vi "daq.io Get Time Series Example.vi"(8 "error in":errorcluster) -> (0 "error out":errorcluster)   [LabVIEW 2013, in "daqio minimal.lvlib"]
doc: "This interactive example demonstrates how to retrieve time series data stored on daq.io in your LabVIEW environment. After connecting, select the device to view data for. Choose a channel to view, select a start and end time to filter data for and choose a time resolution. \n\nMonthly Rollups are very small documents that contain the hourly averages of all measured values.\nDaily Rollups are medium sized documents that contain the measured values averaged to minute data. \nThe Hourly Rollups are documents that store the original resolution with a maximum resolution of 1 Hz. \n\nClick \"Download Data\" to view the selected time frame. \n\nIf Waveform data has been stored on a channel, once you select a channel and filter the start end end time, all existing Waveform documents will be listed below the charting area. Double-click a waveform to download and display it."
uses:
  daqio minimal.lvlib
  _typedefs/exmpl_overlay_mask.ctl
  _typedefs/daqio-rollups-resolution.ctl
  _typedefs/download-2-button.ctl
  _typedefs/daqio-Credentials.ctl
  _typedefs/daqio-Type.ctl
  <vilib>/httpClient/ClientHandle.ctl
  _typedefs/daqio-Device-Specifier.ctl
  <vilib>/Platform/browser.llb/Open URL in Default Browser (string).vi
  <vilib>/httpClient/LabVIEWHTTPClient.lvlib
panel:
  out "overlay mask":T1
  in  "Waveforms":i32(listbox) caption="Waveforms (double-click to view)"
  out "Wfm Graph":waveform(dbl)[](graph) caption="Waveform Graph"
  out "Timeseries Data Graph":cluster{"timestamp":timestamp, "value":dbl}[](graph)
  out "Waveform":string
  in  "Device":u16(ring) items=["DESKTOP_7UDDDR9_LOCALDOMAIN"]
  in  "Download Time Series":T2
  in  "time resolution":T3
  in  "End Time":timestamp
  in  "Start Time":timestamp
  out "selected Channel":string
  in  "Channels":i32(listbox)
  out "Log":string[](array[string])
  in  "Stop":bool
  out "connected to daq.io":bool
  in  "Sign up link":bool caption="Boolean"
  out "Device Key":string
  in  "Log On":bool
  in  "User Name (your email)":string
  in  "Password":string
  # "Get your free account at daq.io first: sign up at"
  # "This Machine"
  # "Select Device to Read Data From"
  # "Device Channel Data"
  # "Select Data Channel"
  # "Specifiy Data to Be Viewed"
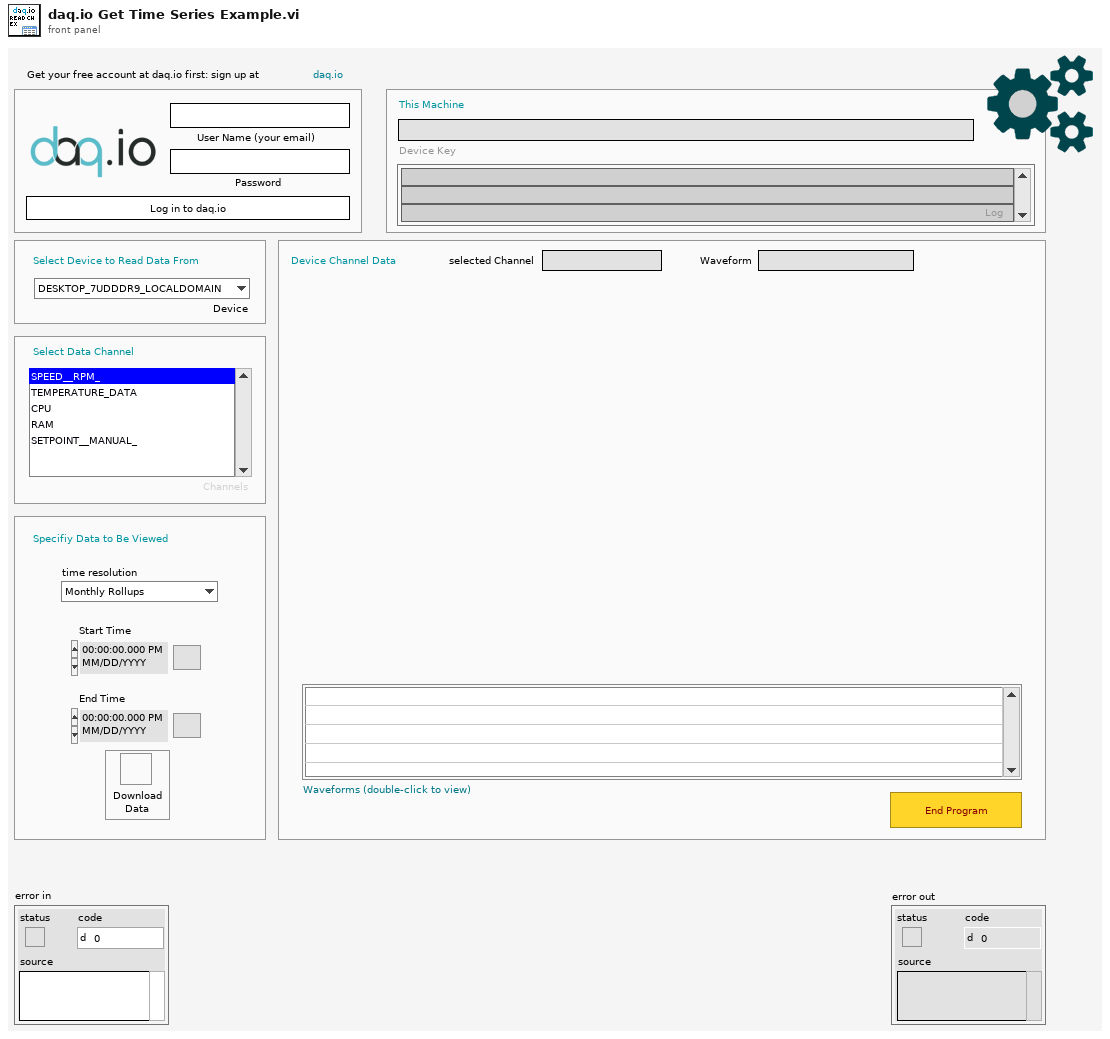
[diagram p1: front panel]
types:
  T1 = typedef "daqio minimal.lvlib/exmpl_overlay_mask.ctl" = bool
  T2 = typedef "daqio minimal.lvlib/download-2-button.ctl" = bool
  T3 = typedef "daqio minimal.lvlib/daqio-rollups-resolution.ctl" = enum16{"Monthly Rollups", "Daily Rollups", "Hourly Rollups (seconds)"}
  T4 = typedef "daqio minimal.lvlib/daqio-Credentials.ctl" = cluster{"User Name (email)":string, "Password":string}
  T5 = typedef "daqio minimal.lvlib/daqio-Device-Specifier.ctl" = cluster{"Device Key":string, "Device Label":string}
  T6 = typedef "daqio minimal.lvlib/daqio-Type.ctl" = cluster{"daq.io ref":T7, "daq.io API Base":string, "Device Key":string, "Account ID":string, "online":bool, "SSL":bool}
  T7 = typedef "LabVIEWHTTPClient.lvlib/ClientHandle.ctl" = refnum<k1>
  T8 = typedef "daqio minimal.lvlib/daqio-Device.ctl" = cluster{"id":string, "label":string, "key":string, "channels":T9[], "tags":cluster{"key":string, "value":string}[], "events":cluster{"id":string, "key":string, "label":string}[], "files":string[], "permissions":cluster{"write":string[], "read":string[]}, "dashboard":string}
  T9 = typedef "daqio minimal.lvlib/daqio-Channels.ctl" = cluster{"key":string, "label":string, "data_type":string, "id":string}
  T10 = typedef "daqio minimal.lvlib/daqio-read-waveform-JSON-header-time.ctl" = cluster{"id":string, "label":string, "channel":string, "device":string, "start_time":timestamp}
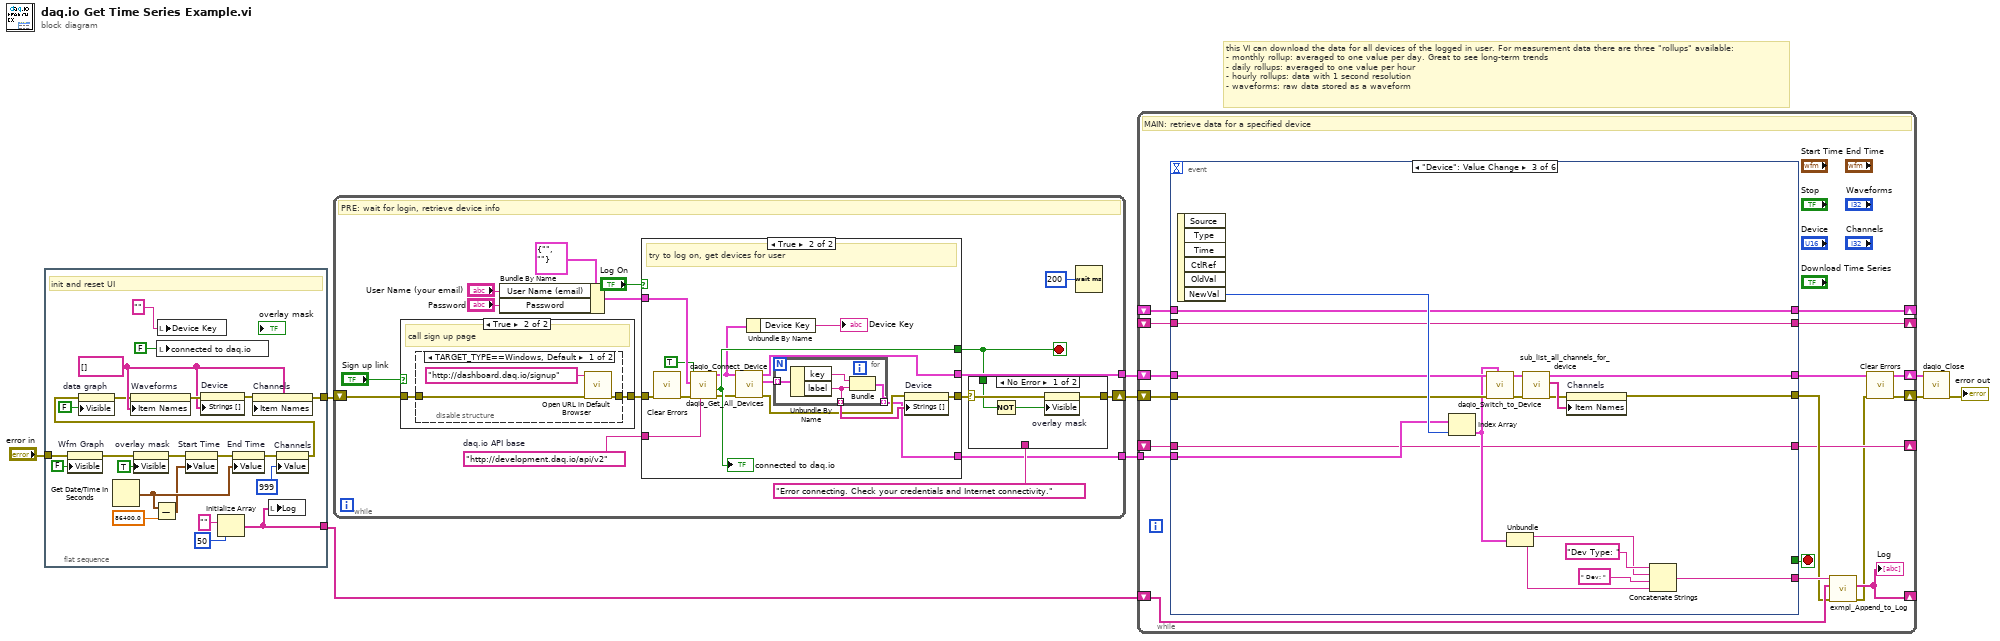
[diagram p0: block diagram]
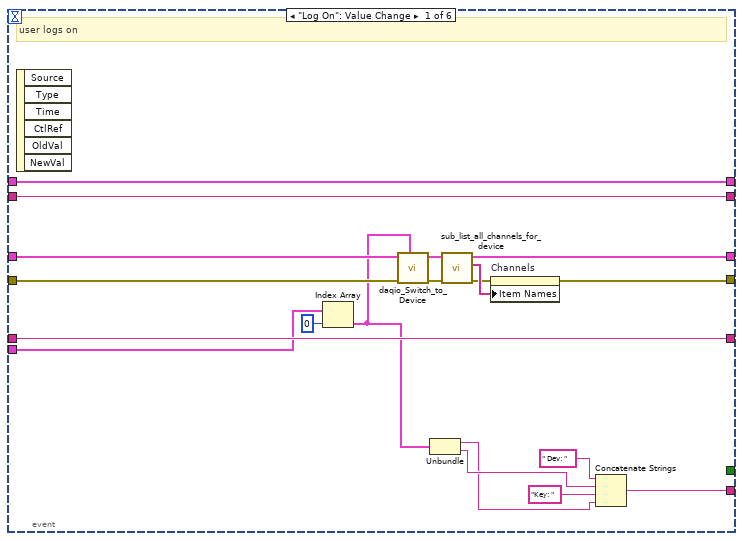
[diagram p2: hidden frame]
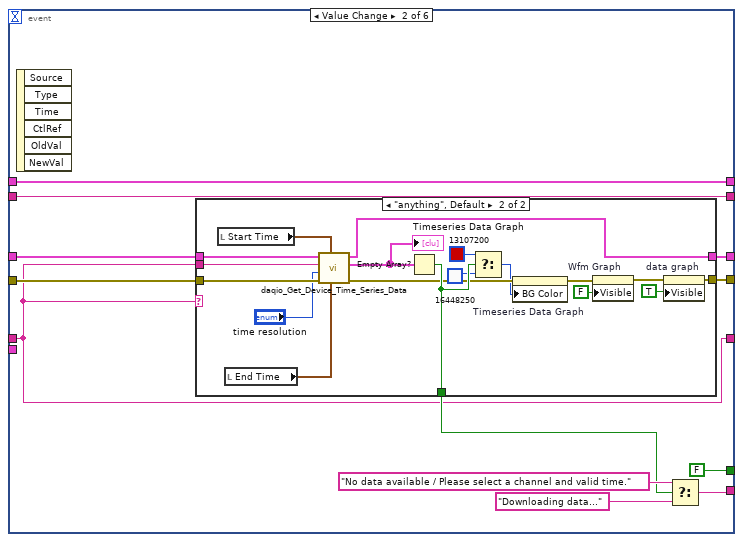
[diagram p3: hidden frame]
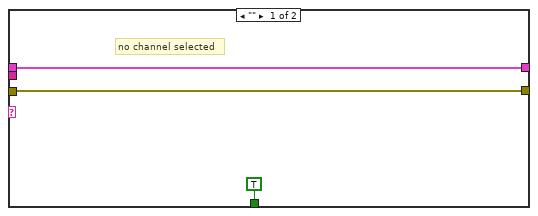
[diagram p4: hidden frame]
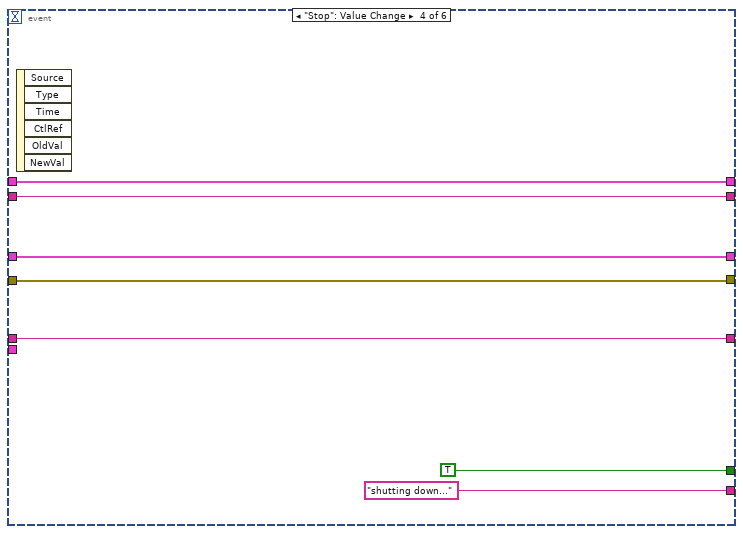
[diagram p5: hidden frame]
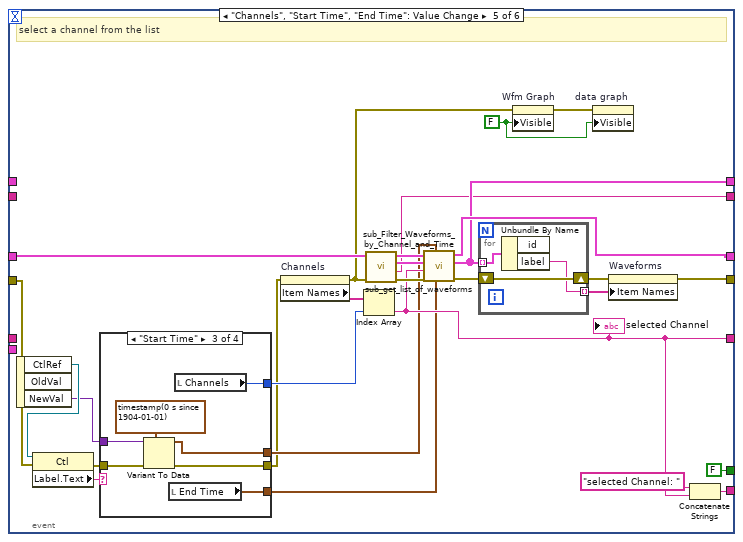
[diagram p6: hidden frame]
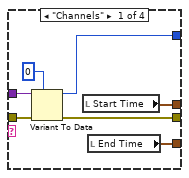
[diagram p7: hidden frame]
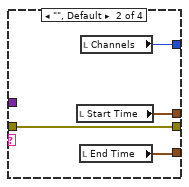
[diagram p8: hidden frame]
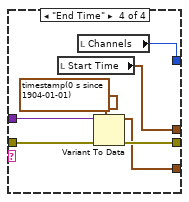
[diagram p9: hidden frame]
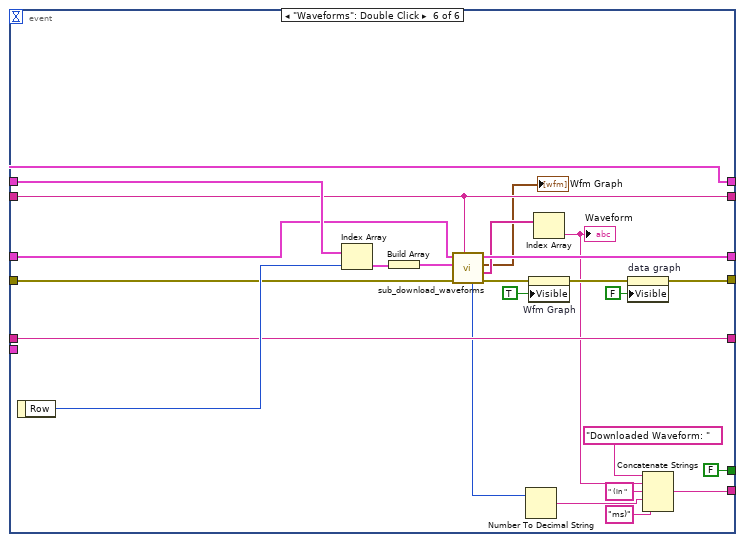
[diagram p10: hidden frame]
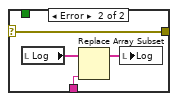
[diagram p11: hidden frame]
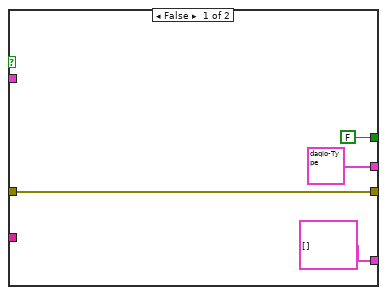
[diagram p14: hidden frame]
diagram:
  # "this VI can download the data for all devices of the logged in user. For measurement data there are three \"rollups\" available: \n- monthly rollup: averaged to one value per day. Great to see long-term trends\n- daily rollups: averaged to one value per hour\n- hourly rollups: data with 1 second resolution\n- waveforms: raw data stored as a waveform"
  n1 = flat-sequence {
    tunnel: [w18] -> w7
    tunnel: "error in" -> [w15]
    tunnel: [w27] -> w3
    frame #0 {
      w16 = string[] [] ("Item Names")
      # "init and reset UI"
      n2 = property on="Wfm Graph" class="WFGraph (strict)"(error in=w15, "Visible"=FALSE) -> (error out=w13:errorcluster)  [unwired: 1 in, 1 out]
      n3 = Get Date/Time In Seconds() -> (seconds since 1Jan1904=w24:timestamp)
      n4 = property on="overlay mask" class="Bool (strict)"(error in=w13, "Visible"=TRUE) -> (error out=w26:errorcluster)  [unwired: 1 in, 1 out]
      n5 = Subtract(x=w24, y=86400.0) -> (x-y=w22:timestamp)
      n6 = local write "connected to daq.io"(FALSE ("connected to daq.io")) -> ()
      n7 = local write "Device Key"("" ("log")) -> ()
      n8 = property on="Start Time" class="AbsTime (strict)"(error in=w26, "Value"=w22) -> (error out=w25:errorcluster)  [unwired: 1 in, 1 out]
      n9 = Initialize Array("" ("log"), 50 ("dimension size")) -> (w27:string[])
      n10 = property on="End Time" class="AbsTime (strict)"(error in=w25, "Value"=w24) -> (error out=w20:errorcluster)  [unwired: 1 in, 1 out]
      n11 = local write "Log"(w27) -> ()
      n12 = property on="Channels" class="LstBox (strict)"(error in=w20, "Value"=999 ("Channels")) -> (error out=w12:errorcluster)  [unwired: 1 in, 1 out]
      n13 = property on="data graph" class="XYGraph (strict)"(error in=w12, "Visible"=FALSE) -> (error out=w11:errorcluster)  [unwired: 1 in, 1 out]
      n14 = property on="Waveforms" class="LstBox (strict)"(error in=w11, "Item Names"=w16) -> (error out=w17:errorcluster)  [unwired: 1 in, 1 out]
      n15 = property on="Device" class="Ring (strict)"(error in=w17, "Strings []"=w16) -> (error out=w19:errorcluster)  [unwired: 1 in, 1 out]
      n16 = property on="Channels" class="LstBox (strict)"(error in=w19, "Item Names"=w16) -> (error out=w18:errorcluster)  [unwired: 1 in, 1 out]
    }
  }
  n17 = while {
    shift-right: [w35] -> w5
    shift-left: w7 -> [w41]
    tunnel: [w43] -> w6
    tunnel: [w34] -> w2
    stop <- w33 stop-if-true
    w38 = "http://development.daq.io/api/v2"  # daq.io API base
    # "PRE: wait for login, retrieve device info"
    n18 = case shown="True" "Sign up link" {
      tunnel: w41 -> [w57 w59]
      tunnel: [w57 w58] -> w40
      frame False {
      }
      frame True {
        # "call sign up page"
        n19 = disable-structure shown="TARGET_TYPE==Windows, Default" {
          disable-tunnel: w59 -> [w61 w63]
          disable-tunnel: [w60 w63] -> w58
          frame condition #0 (active) {
            n20 = call-poly <vilib>:"Open URL in Default Browser.vi"("error in (no error)"=w61, "URL"="http://dashboard.daq.io/signup") -> ("error out"=w60:errorcluster)  [unwired: 4 in, 1 out]
          }
          frame condition #1 {
          }
        }
      }
    }
    n21 = Bundle By Name(cluster=T4 {"User Name (email)"="", "Password"=""} ("daq.io Credentials"), "User Name (email)"="User Name (your email)", "Password"="Password") -> (w42:T4)
    n22 = case shown="True" "Log On" {
      tunnel: [T6 {"daq.io ref"=refnum, "daq.io API Base"="http://dashboard.daq.io/api/v1", "Device Key"="", "Account ID"="", "online"=FALSE, "SSL"=FALSE} ("daq.io type out") w72] -> w43
      tunnel: [w65 w76] -> w36
      tunnel: w40 -> [w65 w82]
      tunnel: w38 -> [_ w81]
      tunnel: w42 -> [_ w80]
      tunnel: [FALSE ("connected successfully?") w79] -> w33
      tunnel: [T5[] [] ("List of Devices") w68] -> w34
      frame False {
      }
      frame True {
        # "try to log on, get devices for user"
        n23 = call <vilib>:"Clear Errors.vi"("error in (no error)"=w82) -> ("error out"=w78:errorcluster)  [unwired: 6 in]
        n24 = call "daqio_Connect_Device.vi"("daq.io API base"=w81, "error in (no error)"=w78, "Credentials"=w80, "Use System Status Event?"=TRUE) -> ("error out"=w75:errorcluster, "connected successfully?"=w79:bool, "daq.io type out"=w74:T6)  [unwired: 5 in]
        "connected to daq.io" <- w79
        n25 = call "daqio_Get_All_Devices.vi"("error in"=w75, "daq.io type in"=w74) -> ("error out"=w70:errorcluster, "Devices"=w73:T8[], "daq.io type out"=w72:T6)  [unwired: 7 in]
        n26 = Unbundle By Name(w74) -> ("Device Key"=→"Device Key":string)
        n27 = for {
          tunnel: w73 -> [w86] mode=indexing
          tunnel: [w85] -> w71 mode=indexing
          tunnel: [w83] -> w68 mode=indexing
          n28 = Unbundle By Name(w86) -> ("key"=w84:string, "label"=w85:string)
          n29 = Bundle("key"=w84, "label"=w85) -> (w83:cluster{"key":string, "label":string})  [unwired: 1 in]
        }
        n30 = property on="Device" class="Ring (strict)"(error in=w70, "Strings []"=w71) -> (error out=w76:errorcluster)  [unwired: 1 in, 1 out]
      }
    }
    n31 = case shown="No Error" w36 {
      selector: w36 -> [w51 w53]
      tunnel: "Error connecting. Check your credentials and Internet connectivity." ("new element/subarray") -> [_ w54]
      tunnel: [w52 w53] -> w35
      tunnel: w33 -> [w50 _]
      frame No Error {
        n32 = Not(x=w50) -> (.not. x?=w49:bool)
        n33 = property on="overlay mask" class="Bool (strict)"(error in=w51, "Visible"=w49) -> (error out=w52:errorcluster)  [unwired: 1 in, 1 out]
      }
      frame Error {
        n34 = local read "Log"() -> (w56:string[])
        n35 = Replace Array Subset(array=w56, new element=w54) -> (w55:string[])  [unwired: 1 in]
        n36 = local write "Log"(w55) -> ()
      }
    }
    n37 = Wait (ms)(milliseconds to wait=u32 200) -> ()  [unwired: 1 out]
  }
  n38 = while {
    shift-right: [w93] -> w9
    shift-left: w5 -> [w99]
    shift-right: [w96] -> w4
    shift-left: w6 -> [w98]
    shift-right: [w103] -> _
    shift-left: w3 -> [w101]
    shift-right: [w95] -> _
    shift-left: _ -> [w94]
    tunnel: w2 -> [w91]
    shift-right: [w90] -> _
    shift-left: _ -> [w89]
    shift-right: [w88] -> _
    shift-left: _ -> [w87]
    stop <- w102 stop-if-true
    # "MAIN: retrieve data for a specified device"
    n39 = event shown="[2] \"Device\": Value Change" {
      selector: _ -> [_ _ _ _ _ _]
      dyn-events: _ -> [_ _ _ _ _ _]
      timeout: _ -> [_ _ _ _ _ _]
      tunnel: [_ FALSE _ TRUE FALSE FALSE] -> w102
      tunnel: [w111 w130 w159 "shutting down..." w206 w242] -> w100
      tunnel: w99 -> [w116 w134 w171 w178 w188 w257]
      tunnel: w98 -> [w117 w133 w172 w177 w205 w256]
      tunnel: [w112 w126 w165 w178 w198 w252] -> w97
      tunnel: [w113 w127 w166 w177 w197 w254] -> w96
      tunnel: [w122 w123 w156 w179 w201 w246] -> w95
      tunnel: w94 -> [w122 w123 w156 w179 _ w246]
      tunnel: w91 -> [w114 _ w173 _ _ _]
      tunnel: [w110 w125 w158 w176 w195 w260] -> w90
      tunnel: w89 -> [w110 w125 w158 w176 _ w260]
      tunnel: [w109 w124 w157 w175 w194 w255] -> w88
      tunnel: w87 -> [w109 w124 w157 w175 _ w255]
      event "Log On": Value Change {
        # "user logs on"
        n40 = event-data() -> ()  [unwired: 1 in, 6 out]
        n41 = Index Array(array=w114, index=0) -> (element=w108:T5)
        n42 = call "daqio_Switch_to_Device.vi"("Device to switch to"=w108, "error in (no error)"=w116, "daq.io type in"=w117) -> ("error out"=w120:errorcluster, "daq.io type out"=w121:T6)  [unwired: 7 in]
        n43 = Unbundle(w108) -> ("Device Key"=w104:string, "Device Label"=w106:string)
        n44 = call "sub_list_all_channels_for_device.vi"("error in (no error)"=w120, "daq.io type in"=w121) -> ("error out"=w118:errorcluster, "List of Channel Keys"=w119:string[], "daq.io type out"=w113:T6)  [unwired: 7 in]
        n45 = property on="Channels" class="LstBox (strict)"(error in=w118, "Item Names"=w119) -> (error out=w112:errorcluster)  [unwired: 1 in, 1 out]
        n46 = Concatenate Strings(" Dev: ", w106, "Key: " ("string"), w104) -> (w111:string)
      }
      event Value Change {
        n47 = event-data() -> ()  [unwired: 1 in, 6 out]
        n48 = case shown="\"anything\", Default" w123 {
          tunnel: w134 -> [w136 w155]
          tunnel: w133 -> [w135 w154]
          tunnel: w123 -> [_ w153]
          tunnel: [TRUE ("empty?") w150] -> w129
          tunnel: [w135 w148] -> w127
          tunnel: [w136 w141] -> w126
          frame "" {
            # "no channel selected"
          }
          frame "anything", Default {
            n49 = local read "Start Time"() -> (w138:timestamp)
            n50 = local read "End Time"() -> (w139:timestamp)
            n51 = call "daqio_Get_Device_Time_Series_Data.vi"("End Time"=w139, "Start Time"=w138, "error in (no error)"=w155, "time resolution"="time resolution", "Channel Key"=w153, "daq.io type in"=w154) -> ("error out"=w149:errorcluster, "Datapoints out"=w151:cluster{"timestamp":timestamp, "value":dbl}[], "daq.io type out"=w148:T6)  [unwired: 3 in]
            "Timeseries Data Graph" <- w151
            n52 = Empty Array?(array=w151) -> (empty?=w150:bool)
            n53 = Select(t=u32 13107200, s=w150, f=u32 16448250) -> (s? t:f=w146:u32)
            n54 = property on="Timeseries Data Graph" class="XYGraph (strict)"(error in=w149, "BG Color"=w146) -> (error out=w144:errorcluster)  [unwired: 1 in, 1 out]
            n55 = property on="Wfm Graph" class="WFGraph (strict)"(error in=w144, "Visible"=FALSE) -> (error out=w140:errorcluster)  [unwired: 1 in, 1 out]
            n56 = property on="data graph" class="XYGraph (strict)"(error in=w140, "Visible"=TRUE) -> (error out=w141:errorcluster)  [unwired: 1 in, 1 out]
          }
        }
        n57 = Select(t="No data available / Please select a channel and valid time.", s=w129, f="Downloading data...") -> (s? t:f=w130:string)
      }
      event "Device": Value Change {
        n58 = event-data() -> ("NewVal"=w174:u16)  [unwired: 1 in, 5 out]
        n59 = Index Array(array=w173, index=w174) -> (element=w162:T5)
        n60 = call "daqio_Switch_to_Device.vi"("Device to switch to"=w162, "error in (no error)"=w171, "daq.io type in"=w172) -> ("error out"=w169:errorcluster, "daq.io type out"=w170:T6)  [unwired: 7 in]
        n61 = Unbundle(w162) -> ("Device Key"=w161:string, "Device Label"=w160:string)
        n62 = call "sub_list_all_channels_for_device.vi"("error in (no error)"=w169, "daq.io type in"=w170) -> ("error out"=w167:errorcluster, "List of Channel Keys"=w168:string[], "daq.io type out"=w166:T6)  [unwired: 7 in]
        n63 = property on="Channels" class="LstBox (strict)"(error in=w167, "Item Names"=w168) -> (error out=w165:errorcluster)  [unwired: 1 in, 1 out]
        n64 = Concatenate Strings("Dev Type: ", w161, " Dev: ", w160) -> (w159:string)
      }
      event "Stop": Value Change {
        n65 = event-data() -> ()  [unwired: 1 in, 6 out]
      }
      event "Channels", "Start Time", "End Time": Value Change {
        w193 = FALSE ("Visible")
        # "select a channel from the list"
        n66 = event-data() -> ("CtlRef"=w190:refnum<vi>, "NewVal"=w187:variant)  [unwired: 1 in, 1 out]
        n67 = property class="Ctl"(reference=w190, error in=w188) -> (error out=w186:errorcluster, "Label.Text"=w189:string)  [unwired: 1 out]
        n68 = case shown="\"Start Time\"" w189 {
          tunnel: w187 -> [w215 _ w225 w233]
          tunnel: w186 -> [w216 w217 w227 w234]
          tunnel: [w213 w220 w222 w231] -> w185
          tunnel: [w212 w218 w224 w230] -> w184
          tunnel: [w211 w219 w223 w228] -> w182
          tunnel: [w210 w217 w221 w232] -> w183
          frame "Channels" {
            n69 = Variant To Data(error in=w216, type=0, Variant=w215) -> (data=w213:i32, error out=w210:errorcluster)
            n70 = local read "Start Time"() -> (w212:timestamp)
            n71 = local read "End Time"() -> (w211:timestamp)
          }
          frame "", Default {
            n72 = local read "Start Time"() -> (w218:timestamp)
            n73 = local read "End Time"() -> (w219:timestamp)
            n74 = local read "Channels"() -> (w220:i32)
          }
          frame "Start Time" {
            n75 = Variant To Data(error in=w227, type=timestamp(0 s since 1904-01-01), Variant=w225) -> (data=w224:timestamp, error out=w221:errorcluster)
            n76 = local read "End Time"() -> (w223:timestamp)
            n77 = local read "Channels"() -> (w222:i32)
          }
          frame "End Time" {
            n78 = local read "Start Time"() -> (w230:timestamp)
            n79 = local read "Channels"() -> (w231:i32)
            n80 = Variant To Data(error in=w234, type=timestamp(0 s since 1904-01-01), Variant=w233) -> (data=w228:timestamp, error out=w232:errorcluster)
          }
        }
        n81 = property on="Channels" class="LstBox (strict)"(error in=w183) -> (error out=w191:errorcluster, "Item Names"=w209:string[])  [unwired: 1 in, 1 out]
        n82 = Index Array(array=w209, index=w185) -> (element=w201:string)
        "selected Channel" <- w201
        n83 = call "sub_get_list_of_waveforms.vi"("error in"=w191, "daq.io type in"=w205) -> ("error out"=w204:errorcluster, "Waveform base URI"=w194:string, "Existing Waveforms"=w203:T10[], "daq.io type out"=w202:T6)  [unwired: 6 in]
        n84 = call "sub_Filter_Waveforms_by_Channel_and_Time.vi"("End Time"=w182, "Start Time"=w184, "error in"=w204, "Channel Key"=w201, "Waveforms in"=w203, "daq.io type in"=w202) -> ("error out"=w199:errorcluster, "Filtered Waveforms out"=w195:T10[], "daq.io type out"=w197:T6)  [unwired: 3 in]
        n85 = for {
          tunnel: w195 -> [w236] mode=indexing
          shift-right: [w237] -> w200
          shift-left: w199 -> [w237]
          tunnel: [w235] -> w196 mode=indexing
          n86 = Unbundle By Name(w236) -> ("label"=w235:string)  [unwired: 1 out]
        }
        n87 = property on="Wfm Graph" class="WFGraph (strict)"(error in=w191, "Visible"=w193) -> (error out=w192:errorcluster)  [unwired: 1 in, 1 out]
        n88 = property on="data graph" class="XYGraph (strict)"(error in=w192, "Visible"=w193) -> ()  [unwired: 1 in, 2 out]
        n89 = property on="Waveforms" class="LstBox (strict)"(error in=w200, "Item Names"=w196) -> (error out=w198:errorcluster)  [unwired: 1 in, 1 out]
        n90 = Concatenate Strings("selected Channel: ", w201) -> (w206:string)
      }
      event "Waveforms": Double Click {
        n91 = event-data() -> ("Row"=w261:i32)  [unwired: 1 in]
        n92 = Index Array(array=w260, index=w261) -> (element=w259:T10)
        n93 = Build Array(w259) -> (w258:T10[])
        n94 = call "sub_download_waveforms.vi"("Waveform base URI"=w255, "error in"=w257, "Filtered Waveforms in"=w258, "daq.io type in"=w256) -> ("error out"=w249:errorcluster, "Waveform Labels out"=w251:string[], "Waveform Data out"=→"Wfm Graph":waveform(dbl)[], "daq.io type out"=w254:T6, "time elapsed (ms)"=w241:u32)  [unwired: 3 in]
        n95 = Number To Decimal String(number=w241) -> (decimal integer string=w239:string)  [unwired: 1 in]
        n96 = property on="Wfm Graph" class="WFGraph (strict)"(error in=w249, "Visible"=TRUE) -> (error out=w248:errorcluster)  [unwired: 1 in, 1 out]
        n97 = Index Array(array=w251) -> (element=w243:string)  [unwired: 1 in]
        "Waveform" <- w243
        n98 = property on="data graph" class="XYGraph (strict)"(error in=w248, "Visible"=FALSE) -> (error out=w252:errorcluster)  [unwired: 1 in, 1 out]
        n99 = Concatenate Strings("Downloaded Waveform: ", w243, " (in " ("string"), w239, "ms)" ("string")) -> (w242:string)
      }
    }
    n100 = call "exmpl_Append_to_Log.vi"("error in (no error)"=w97, "Log Array in"=w101, "Log Message"=w100) -> ("error out"=w92:errorcluster, "Log Array out"=w103:string[])  [unwired: 7 in]
    "Log" <- w103
    n101 = call <vilib>:"Clear Errors.vi"("error in (no error)"=w92) -> ("error out"=w93:errorcluster)  [unwired: 6 in]
  }
  n102 = call "daqio_Close.vi"("error in (no error)"=w9, "daq.io type"=w4) -> ("error out"=→"error out":errorcluster)  [unwired: 9 in]
